vi "test Configuration Files Errors.vi"(8 "error in":errorcluster, 11 "TestCase in":refnum<class "Scripting.lvclass">) -> (0 "error out":errorcluster, 3 "TestCase out":refnum<class "Scripting.lvclass">)   [LabVIEW 2020, in "Scripting.lvclass"]
uses:
  Scripting.lvclass
  C:/Git/niveristand-custom-device-testing-tools/VeriStandScriptingTestCase/VeriStandScriptingTestCase.lvclass
  niveristand-custom-device-testing-tools/VeriStandScriptingTestCase/VeriStandScriptingTestCase.lvclass/VeriStandScriptingTestCase.ctl
  niveristand-custom-device-testing-tools/VeriStandScriptingTestCase/Read Target.vi
  Scripting/Constants.vi
  NationalInstruments.VeriStand.SystemDefinitionAPI
  <vilib>/addons/_JKI Toolkits/VI Tester/TestCase.llb/TestCase.lvclass
  Scripting/Ballard MIL-STD-1553 Scripting.lvlib
  niveristand-custom-device-testing-tools/VeriStandTestUtilities/VeriStandTestUtilities.lvlib
  C:/Program Files (x86)/National Instruments/LabVIEW 2020/vi.lib/addons/_JKI Toolkits/VI Tester/TestCase.llb/TestCase.lvclass
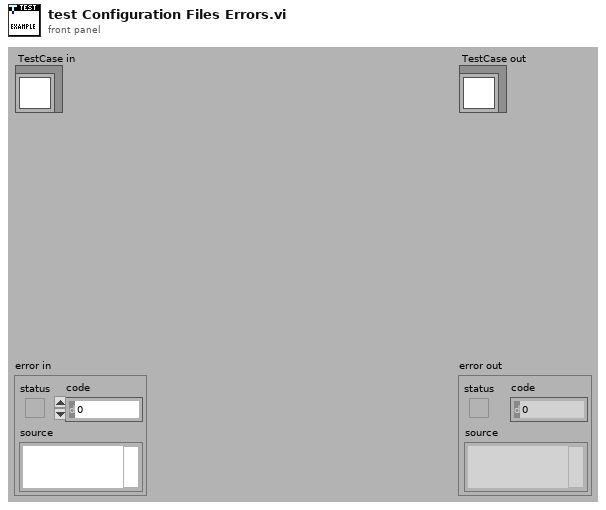
[diagram p1: front panel]
types:
  T1 = typedef "Custom Device API.lvlib/Custom Device Item Ref.ctl" = u64
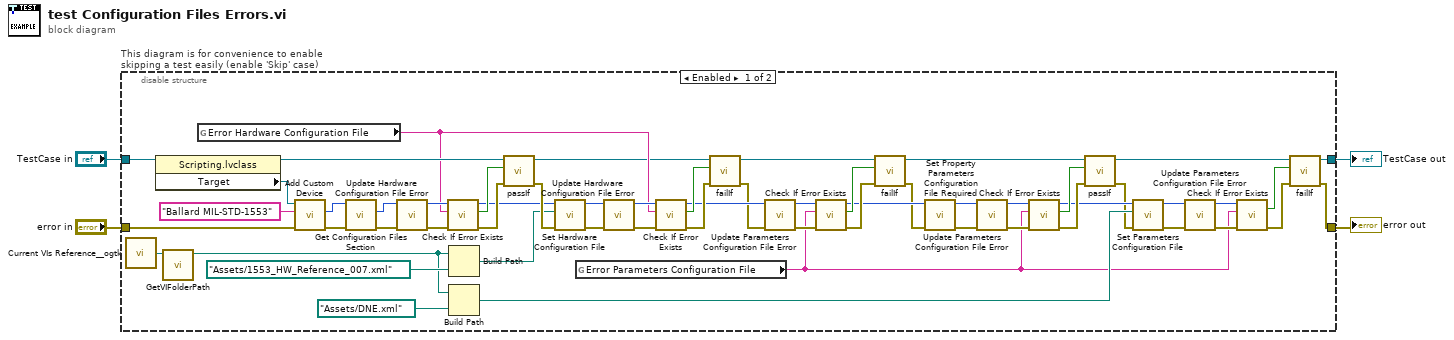
[diagram p0: block diagram]
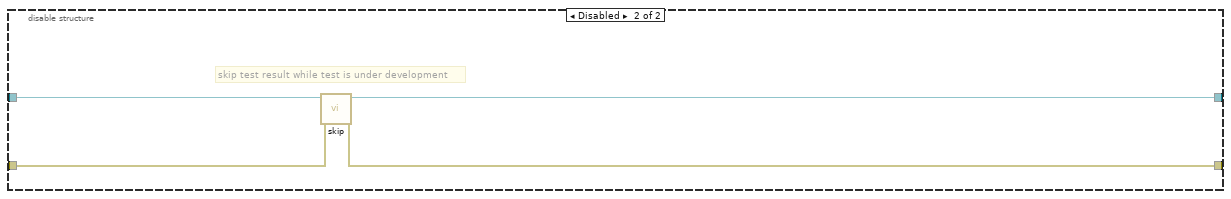
[diagram p2: hidden frame]
diagram:
  n1 = disable-structure "This diagram is for convenience to enable skipping a test easily (enable 'Skip' case)" shown="Enabled" {
    disable-tunnel: "TestCase in" -> [w59 w65]
    disable-tunnel: [w5 w63] -> w1
    disable-tunnel: [w6 w64] -> w3
    disable-tunnel: "error in" -> [w61 w62]
    frame Enabled {
      n2 = call <userlib>:"Current VIs Reference__ogtk.vi"() -> ("Current VI's reference"=w57:refnum<vi>)  [unwired: 5 in]
      n3 = property class="Scripting.lvclass"(reference=w59) -> (reference out=w52:refnum<class "Scripting.lvclass">, "Target"=w58:refnum<k24>)  [unwired: 1 in, 1 out]
      n4 = call "GetVIFolderPath.vi"("VI Reference in"=w57) -> ("VI Folder Path out"=w17:path)  [unwired: 9 in, 1 out]
      n5 = global read "Constants.vi" "Error Hardware Configuration File"() -> (w44:string)
      n6 = call "Add Custom Device.vi"("error in"=w61, "name"="Ballard MIL-STD-1553", "target in"=w58) -> ("error out"=w32:errorcluster, "Ballard MIL-STD 1553 custom device"=w33:T1)  [unwired: 6 in, 1 out]
      n7 = call "Get Configuration Files Section.vi"("error in"=w32, "custom device in"=w33) -> ("error out"=w31:errorcluster, "configuration files section"=w30:T1)  [unwired: 7 in, 1 out]
      n8 = call "Update Hardware Configuration File Error.vi"("error in"=w31, "configuration files ref in"=w30) -> ("error out"=w54:errorcluster, "configuration files ref out"=w53:T1)  [unwired: 8 in]
      n9 = call "Check If Error Exists.vi"("error in"=w54, "error key"=w44, "section ref in"=w53) -> ("error out"=w51:errorcluster, "error exists?"=w50:bool, "section ref out"=w49:T1)  [unwired: 6 in]
      n10 = Build Path(base path=w17, name or relative path=path "Assets/1553_HW_Reference_007.xml" ("hardware configuration file path")) -> (appended path=w18:path)
      n11 = Build Path(base path=w17, name or relative path=path "Assets/DNE.xml" ("hardware configuration file path")) -> (appended path=w15:path)
      n12 = call-dynamic "passIf.vi"("error in (no error)"=w51, "pass"=w50, "TestCase in"=w52) -> ("error out"=w55:errorcluster, "TestCase out"=w43:refnum<class "Scripting.lvclass">)  [unwired: 7 in]
      n13 = call "Set Hardware Configuration File.vi"("error in"=w55, "hardware configuration file path"=w18, "Ballard MIL-STD 1553 custom device in"=w49) -> ("error out"=w45:errorcluster, "Ballard MIL-STD 1553 custom device out"=w46:T1)  [unwired: 7 in]
      n14 = global read "Constants.vi" "Error Parameters Configuration File"() -> (w8:string)
      n15 = call "Update Hardware Configuration File Error.vi"("error in"=w45, "configuration files ref in"=w46) -> ("error out"=w47:errorcluster, "configuration files ref out"=w48:T1)  [unwired: 8 in]
      n16 = call "Check If Error Exists.vi"("error in"=w47, "error key"=w44, "section ref in"=w48) -> ("error out"=w42:errorcluster, "error exists?"=w41:bool, "section ref out"=w40:T1)  [unwired: 6 in]
      n17 = call-dynamic "failIf.vi"("error in (no error)"=w42, "fail"=w41, "TestCase in"=w43) -> ("error out"=w39:errorcluster, "TestCase out"=w34:refnum<class "Scripting.lvclass">)  [unwired: 7 in]
      n18 = call "Update Parameters Configuration File Error.vi"("error in"=w39, "configuration files ref in"=w40) -> ("error out"=w38:errorcluster, "configuration files ref out"=w37:T1)  [unwired: 8 in]
      n19 = call "Check If Error Exists.vi"("error in"=w38, "error key"=w8, "section ref in"=w37) -> ("error out"=w36:errorcluster, "error exists?"=w35:bool, "section ref out"=w29:T1)  [unwired: 6 in]
      n20 = call-dynamic "failIf.vi"("error in (no error)"=w36, "fail"=w35, "TestCase in"=w34) -> ("error out"=w28:errorcluster, "TestCase out"=w23:refnum<class "Scripting.lvclass">)  [unwired: 7 in]
      n21 = call "Set Property Parameters Configuration File Required.vi"("error in"=w28, "configuration files ref"=w29) -> ("error out"=w24:errorcluster, "configuration files ref out"=w25:T1)  [unwired: 8 in]
      n22 = call "Update Parameters Configuration File Error.vi"("error in"=w24, "configuration files ref in"=w25) -> ("error out"=w26:errorcluster, "configuration files ref out"=w27:T1)  [unwired: 8 in]
      n23 = call "Check If Error Exists.vi"("error in"=w26, "error key"=w8, "section ref in"=w27) -> ("error out"=w22:errorcluster, "error exists?"=w21:bool, "section ref out"=w14:T1)  [unwired: 6 in]
      n24 = call-dynamic "passIf.vi"("error in (no error)"=w22, "pass"=w21, "TestCase in"=w23) -> ("error out"=w13:errorcluster, "TestCase out"=w10:refnum<class "Scripting.lvclass">)  [unwired: 7 in]
      n25 = call "Set Parameters Configuration File.vi"("error in"=w13, "parameters configuration file path"=w15, "Ballard MIL-STD 1553 custom device in"=w14) -> ("error out"=w11:errorcluster, "Ballard MIL-STD 1553 custom device out"=w12:T1)  [unwired: 7 in]
      n26 = call "Update Parameters Configuration File Error.vi"("error in"=w11, "configuration files ref in"=w12) -> ("error out"=w20:errorcluster, "configuration files ref out"=w19:T1)  [unwired: 8 in]
      n27 = call "Check If Error Exists.vi"("error in"=w20, "error key"=w8, "section ref in"=w19) -> ("error out"=w7:errorcluster, "error exists?"=w9:bool)  [unwired: 6 in, 1 out]
      n28 = call-dynamic "failIf.vi"("error in (no error)"=w7, "fail"=w9, "TestCase in"=w10) -> ("error out"=w6:errorcluster, "TestCase out"=w5:refnum<class "Scripting.lvclass">)  [unwired: 7 in]
    }
    frame Disabled {
      # "skip test result while test is under development"
      n29 = call <vilib>:"skip.vi"("error in (no error)"=w62, "TestCase in"=w65) -> ("error out"=w64:errorcluster, "TestCase out"=w63:refnum<class "Scripting.lvclass">)  [unwired: 8 in]
    }
  }
  "error out" <- w3
  "TestCase out" <- w1
